vi "题目三.vi"() -> ()   [LabVIEW 2017]
uses:
  <vilib>/measure/NI_MABase.lvlib
panel:
  out "Y":dbl[](array[numeric])
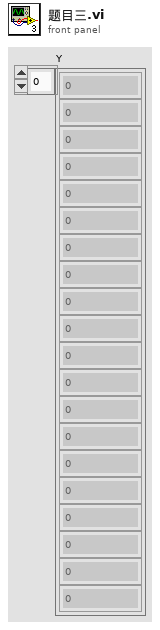
[diagram p1: front panel]
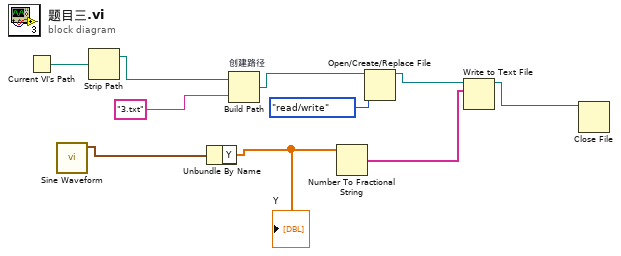
[diagram p0: block diagram]
diagram:
  n1 = Current VI's Path() -> (path=w9:path)
  n2 = call <vilib>:"Sine Waveform.vi"() -> ("signal out"=w10:waveform(dbl))  [unwired: 10 in, 1 out]
  n3 = Strip Path(path=w9) -> (stripped path=w8:path)  [unwired: 1 out]
  n4 = Unbundle By Name(w10) -> ("Y"=w3:dbl[])
  "Y" <- w3
  n5 = Build Path "创建路径"(base path=w8, name or relative path="3.txt" ("名称或相对路径")) -> (appended path=w6:path)
  n6 = Number To Fractional String(number=w3) -> (F-format string=w2:string[])  [unwired: 3 in]
  n7 = Open/Create/Replace File(file path (use dialog)=w6, access (0:read/write)=enum16{"read/write", "read-only", "write-only"}."read/write" ("权限(0:read/write)")) -> (refnum out=w4:refnum<file>)  [unwired: 4 in, 2 out]
  n8 = Write to Text File(file (use dialog)=w4, text=w2) -> (refnum out=w1:refnum<file>)  [unwired: 2 in, 2 out]
  n9 = Close File(refnum=w1) -> ()  [unwired: 1 in, 2 out]
